vi "TCP_Server.vi"() -> ()   [LabVIEW 2020]
panel:
  in  "Data tx":string
  in  "stop":bool
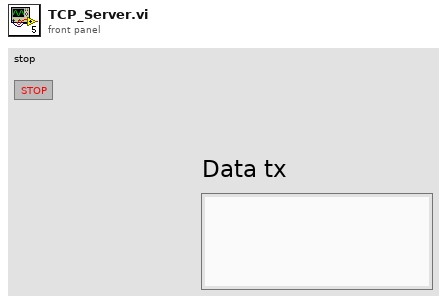
[diagram p1: front panel]
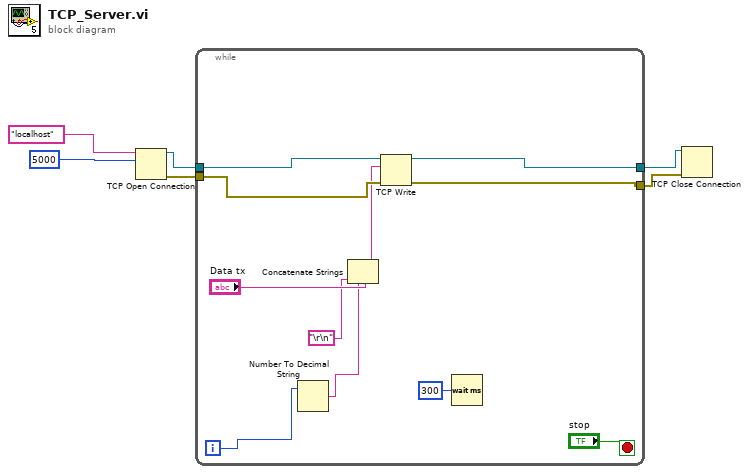
[diagram p0: block diagram]
diagram:
  n1 = TCP Open Connection(address="localhost", remote port or service name=u16 5000) -> (connection ID=w5:refnum<k5>, error out=w4:errorcluster)  [unwired: 3 in]
  n2 = while {
    tunnel: w5 -> [w16]
    tunnel: w4 -> [w15]
    tunnel: [w14] -> w3
    tunnel: [w7] -> w1
    i -> [w12]
    stop <- "stop" stop-if-true
    n3 = Number To Decimal String(number=w12) -> (decimal integer string=w10:string)  [unwired: 1 in]
    n4 = Concatenate Strings("Data tx", w10, "\r\n") -> (w8:string)
    n5 = TCP Write(connection ID=w16, data in=w8, error in (no error)=w15) -> (connection ID out=w14:refnum<k5>, error out=w7:errorcluster)  [unwired: 1 in, 1 out]
    n6 = Wait (ms)(milliseconds to wait=u32 300) -> ()  [unwired: 1 out]
  }
  n7 = TCP Close Connection(connection ID=w3, error in (no error)=w1) -> ()  [unwired: 1 in, 2 out]
